vi "Plot Frequency Response - cascade.vi"(0 "samples":i32=201, 1 "use dB":bool, 2 "IIR Filter Cluster":T1, 4 "unwrap":bool) -> (5 "Magnitude":cluster{dbl[], dbl[]}(graph), 6 "Phase":cluster{dbl[], dbl[]}(graph), 7 "Group Delay":cluster{dbl[], dbl[]}(graph))   [LabVIEW 2016]
doc: "Plot the frequency response of a filter described by its cascade-form IIR filter cluster."
uses:
  <vilib>/Analysis/1siggen.llb/Ramp Pattern by Samples.vi
  <vilib>/Analysis/polynomials.llb/1D Polynomial Evaluation (CDB).vi
  <vilib>/Analysis/NI_AALBase.lvlib
  <vilib>/Analysis/NI_AALPro.lvlib
panel:
  # "freqz_cascade.vi"
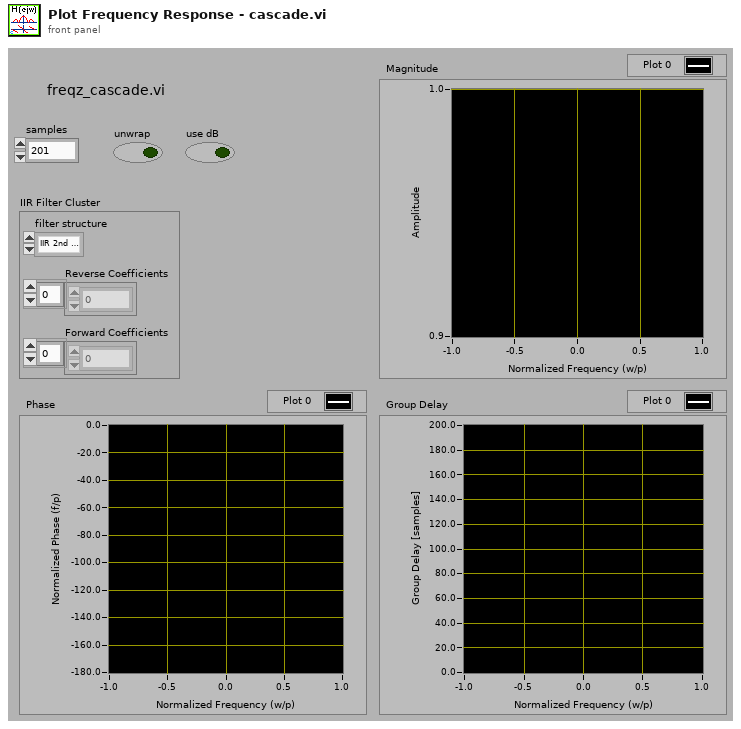
[diagram p1: front panel]
types:
  T1 = cluster{"filter structure":enum32{"IIR 2nd Order", "IIR 4th Order"}, "Reverse Coefficients":dbl[], "Forward Coefficients":dbl[]}
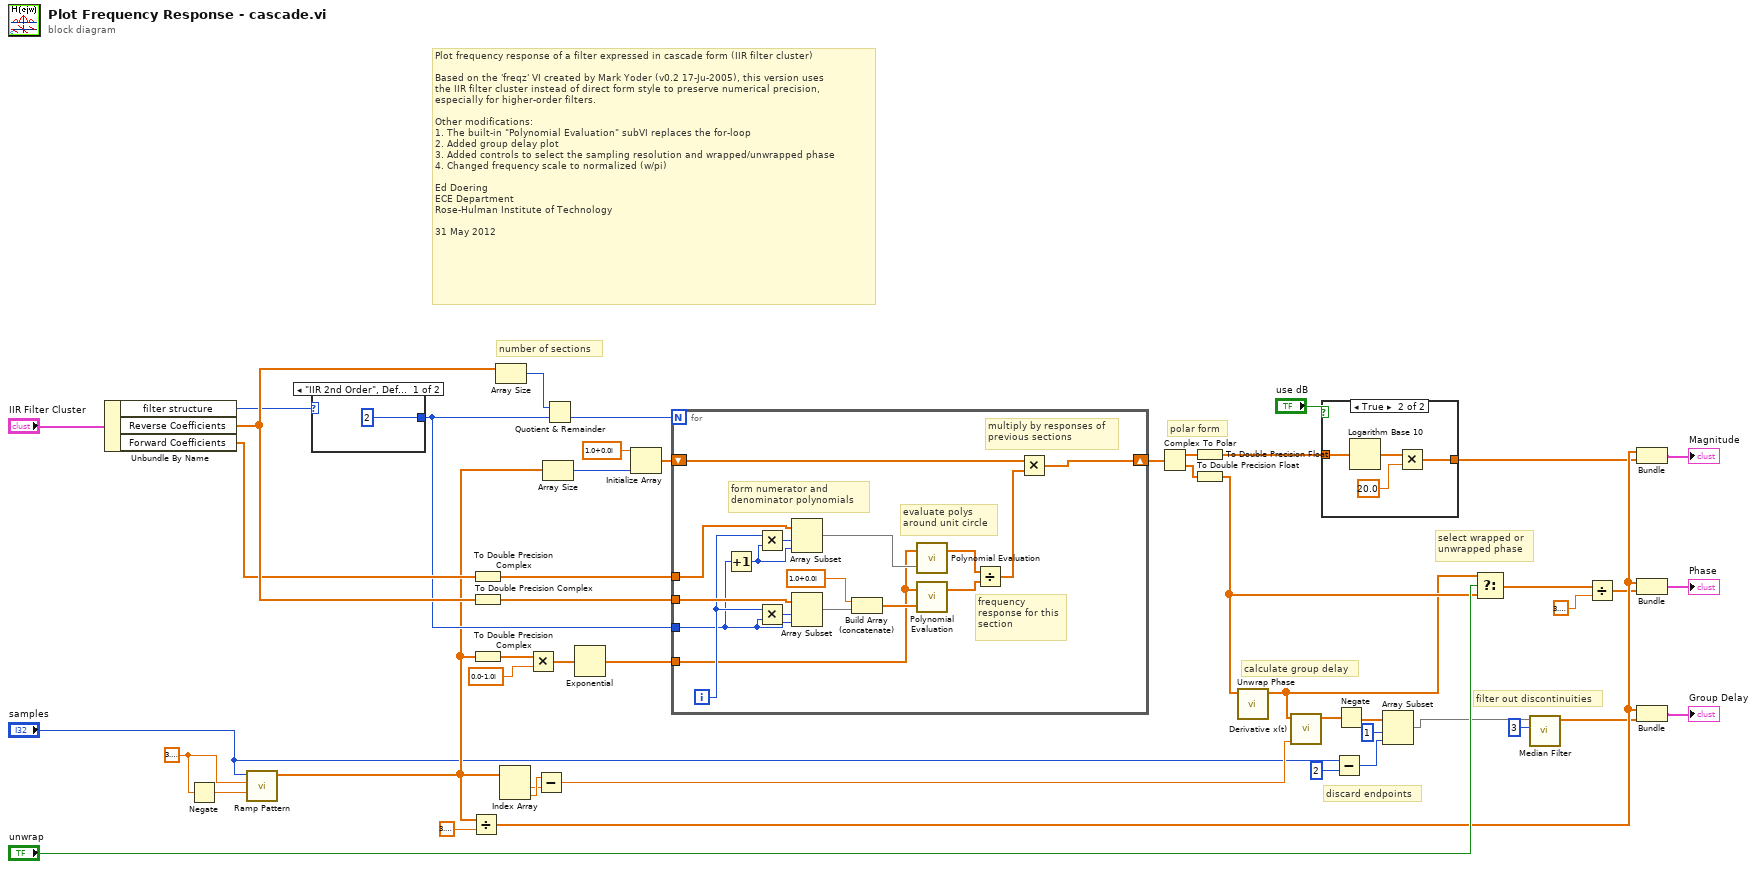
[diagram p0: block diagram]
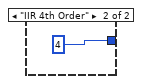
[diagram p3: hidden frame]
diagram:
  w47 = 3.141592653589793
  # "filter out discontinuities"
  # "discard endpoints"
  # "polar form"
  # "select wrapped or\nunwrapped phase"
  # "calculate group delay"
  # "Plot frequency response of a filter expressed in cascade form (IIR filter cluster)\n\nBased on the 'freqz' VI created by Mark Yoder (v0.2 17-Ju-2005), this version uses\nthe IIR filter cluster instead of direct form style to preserve numerical precision,\nespecially for higher-order filters.\n\nOther modifications:\n1. The built-in \"Polynomial Evaluation\" subVI replaces the for-loop\n2. Added group delay plot\n3. Added controls to select the sampling resolution and wrapped/unwrapped phase\n4. Changed frequency scale to normalized (w/pi)\n\nEd Doering\nECE Department\nRose-Hulman Institute of Technology\n\n31 May 2012"
  # "number of sections"
  n1 = Unbundle By Name("IIR Filter Cluster") -> ("filter structure"=w23:enum32{"IIR 2nd Order", "IIR 4th Order"}, "Reverse Coefficients"=w41:dbl[], "Forward Coefficients"=w40:dbl[])
  n2 = Negate(x=w47) -> (-x=w48:dbl)
  n3 = call-poly <vilib>:"Ramp Pattern.vi"("start"=w48, "end"=w47, "samples"="samples") -> ("Ramp Pattern"=w21:dbl[])  [unwired: 7 in, 1 out]
  n4 = case shown="\"IIR 2nd Order\", Default" w23 {
    tunnel: [2 ("y") 4 ("y")] -> w22
    frame "IIR 2nd Order", Default {
    }
    frame "IIR 4th Order" {
    }
  }
  n5 = Divide(x=w21, y=3.141592653589793) -> (x/y=w16:dbl[])
  n6 = To Double Precision Complex(1:w40) -> (0:w44:cdb[])
  n7 = To Double Precision Complex(1:w41) -> (0:w43:cdb[])
  n8 = To Double Precision Complex(1:w21) -> (0:w37:cdb[])
  n9 = Array Size(array=w41) -> (size(s)=w31:i32)
  n10 = Index Array(array=w21) -> (element #1=w26:dbl, element #2=w27:dbl)  [unwired: 2 in]
  n11 = Multiply(x=w37, y=cdb 0.0-1.0i) -> (x*y=w39:cdb[])
  n12 = Subtract(x=w27, y=w26) -> (x-y=w25:dbl)
  n13 = Array Size(array=w21) -> (size(s)=w35:i32)
  n14 = Quotient & Remainder(x=w31, y=w22) -> (floor(x/y)=w30:i32)  [unwired: 1 out]
  n15 = Exponential(1:w39) -> (0:w36:cdb[])
  n16 = Initialize Array(cdb 1.0+0.0i ("dimension size"), w35) -> (w33:cdb[])
  n17 = for {
    N: w30 -> [_]
    tunnel: w44 -> [w64]
    tunnel: w43 -> [w61]
    tunnel: w36 -> [w56]
    shift-right: [w53] -> w32
    shift-left: w33 -> [w55]
    tunnel: w22 -> [w51]
    i -> [w57]
    # "multiply by responses of\nprevious sections"
    # "frequency\nresponse for this\nsection"
    # "evaluate polys\naround unit circle"
    # "form numerator and\ndenominator polynomials"
    n18 = Increment(x=w51) -> (x+1=w52:i32)
    n19 = Multiply(x=w57, y=w52) -> (x*y=w65:i32)
    n20 = Multiply(x=w57, y=w51) -> (x*y=w62:i32)
    n21 = Array Subset(array=w64, index=w65, length=w52) -> (w63:cdb[])
    n22 = Array Subset(array=w61, index=w62, length=w51) -> (w59:cdb[])
    n23 = Build Array (concatenate)(cdb 1.0+0.0i ("element"), w59) -> (w58:cdb[])
    n24 = call-poly <vilib>:"Polynomial Evaluation.vi"("P(x)"=w63, "A"=w56) -> ("P(A)"=w67:cdb[])  [unwired: 1 out]
    n25 = call-poly <vilib>:"Polynomial Evaluation.vi"("P(x)"=w58, "A"=w56) -> ("P(A)"=w66:cdb[])  [unwired: 1 out]
    n26 = Divide(x=w67, y=w66) -> (x/y=w54:cdb[])
    n27 = Multiply(x=w55, y=w54) -> (x*y=w53:cdb[])
  }
  n28 = Complex To Polar(r * e^(i*theta)=w32) -> (r=w46:dbl[], theta=w45:dbl[])
  n29 = To Double Precision Float(number=w46) -> (double precision float=w13:dbl[])
  n30 = To Double Precision Float(number=w45) -> (double precision float=w28:dbl[])
  n31 = call <vilib>:"Unwrap Phase.vi"("Phase"=w28) -> ("Unwrapped Phase"=w19:dbl[])  [unwired: 9 in, 1 out]
  n32 = call <vilib>:"Derivative x(t).vi"("dt"=w25, "X"=w19) -> ("dX/dt"=w24:dbl[])  [unwired: 8 in, 1 out]
  n33 = case shown="True" "use dB" {
    tunnel: w13 -> [w68 w70]
    tunnel: [w68 w69] -> w12
    frame False {
    }
    frame True {
      n34 = Logarithm Base 10(1:w70) -> (0:w71:dbl[])
      n35 = Multiply(x=w71, y=20.0) -> (x*y=w69:dbl[])
    }
  }
  n36 = Subtract(x="samples", y=2) -> (x-y=w9:i32)
  n37 = Negate(x=w24) -> (-x=w6:dbl[])
  n38 = Array Subset(array=w6, index=1, length=w9) -> (w11:dbl[])
  n39 = Select(t=w19, s="unwrap", f=w28) -> (s? t:f=w2:dbl[])
  n40 = call <vilib>:"Median Filter.vi"("left rank"=3, "X"=w11) -> ("Filtered X"=w5:dbl[])  [unwired: 8 in, 1 out]
  n41 = Divide(x=w2, y=3.141592653589793) -> (x/y=w1:dbl[])
  n42 = Bundle(w16, w12) -> (→"Magnitude":cluster{dbl[], dbl[]})  [unwired: 1 in]
  n43 = Bundle(w16, w1) -> (→"Phase":cluster{dbl[], dbl[]})  [unwired: 1 in]
  n44 = Bundle(w16, "Filtered X"=w5) -> (→"Group Delay":cluster{dbl[], "Filtered X":dbl[]})  [unwired: 1 in]
